vi "Close Multiple Channel.vi"(0 "VISA resource name":refnum<visa-resource-name>, 5 "Channel List (101,103:105)":string="101,103:105", 11 "error in (no error)":errorcluster) -> (4 "VISA resource name out":refnum<visa-resource-name>, 15 "error out":errorcluster)   [LabVIEW 2020, in "Keithley 27XX.lvlib"]
doc: "This VI will close channel(s) specified in the list. Unlisted channels are not affected."
uses:
  Keithley 27XX.lvlib
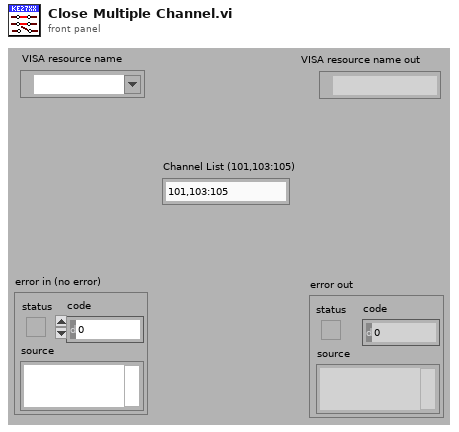
[diagram p1: front panel]
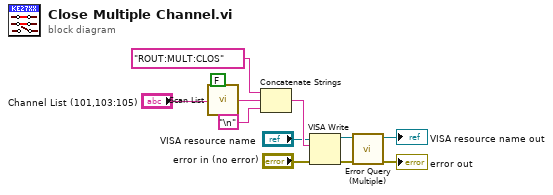
[diagram p0: block diagram]
diagram:
  n1 = call "Scan List.vi"("Add Comma (True)"=FALSE ("Comma? (True)"), "Scan List (Empty)"="Channel List (101,103:105)") -> ("Scan List Out"=w10:string)  [unwired: 13 in]
  n2 = Concatenate Strings("ROUT:MULT:CLOS", w10, "\n") -> (w9:string)
  n3 = VISA Write(VISA resource name="VISA resource name", write buffer=w9, error in (no error)="error in (no error)") -> (VISA resource name out=w5:refnum<visa-resource-name>, error out=w4:errorcluster)  [unwired: 1 out]
  n4 = call "Error Query (Multiple).vi"("VISA resource name"=w5, "error in (no error)"=w4) -> ("VISA resource name out"=→"VISA resource name out":refnum<visa-resource-name>, "error out"=→"error out":errorcluster)  [unwired: 10 in, 2 out]
